vi "authorization.vi"() -> (3 "header":cluster{"header":string, "value":string}={"header"="Content-Type", "value"="application/json"})   [LabVIEW 2015, in "lv-dropbox.lvlib"]
uses:
  lv-dropbox.lvlib
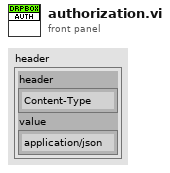
[diagram p1: front panel]
types:
  T1 = typedef "lv-dropbox.lvlib/authorization.ctl" = cluster{"authorization":string, "expire":timestamp}
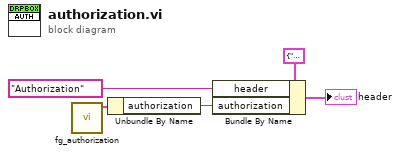
[diagram p0: block diagram]
diagram:
  n1 = call "fg_authorization.vi"() -> ("authorization out"=w5:T1)  [unwired: 10 in, 1 out]
  n2 = Unbundle By Name(w5) -> ("authorization"=w2:string)
  n3 = Bundle By Name(cluster=cluster{"header":string, "authorization":string} {"header"="", "authorization"=""}, "header"="Authorization", "authorization"=w2) -> (→"header":cluster{"header":string, "authorization":string})
